vi "RampVoltagewithDDSv6.vi"() -> ()   [LabVIEW 2016]
uses:
  <vilib>/DAQmx/write.llb/DAQmx Write (Digital 1D Wfm NChan NSamp).vi
  <vilib>/DAQmx/write.llb/DAQmx Write (Analog 2D DBL NChan NSamp).vi
  <vilib>/DAQmx/create/channels.llb/DAQmx Create Channel (AO-Voltage-Basic).vi
  <vilib>/Waveform/DWDTOps.llb/DWDT Boolean Array to Digital.vi
  <vilib>/DAQmx/create/channels.llb/DAQmx Create Channel (DO-Digital Output).vi
  <vilib>/DAQmx/configure/timing.llb/DAQmx Timing (Sample Clock).vi
  <vilib>/DAQmx/configure/trigger.llb/DAQmx Start Trigger (Digital Edge).vi
  <vilib>/Waveform/DWDTOps.llb/DWDT Uncompress Digital.vi
  <vilib>/DAQmx/miscellaneous.llb/DAQmx Fill In Error Info.vi
  <vilib>/Waveform/DTblOps.llb/DTbl Digital to Analog.vi
  <resource>/objmgr/daqmx.rc
panel:
  out "Digital Output":cluster{i32, dbl, dbl[][]}(graph)={0, 0.0001, [[5.0, 5.0, 5.0, 5.0, 5.0, 0.0, 0.0, 0.0, 0.0, 0.0, 0.0, 0.0, 0.0, 0.0, 0.0, 0.0, 0.0, 0.0, 0.0, 0.0, 0.0, 0.0, 0.0, 0.0, 0.0, 5.0, 5.0, 5.0, 5.0, 5.0, 5.0, 5.0, 5.0, 5.0, 5.0, 5.0, 5.0, 5.0, 5.0, 5.0, 5.0, 5.0, 5.0, 5.0, 5.0, 0.0, 0.0, 0.0, 0.0, 0.0, 0.0, 0.0, 0.0, 0.0, 0.0, 0.0, 0.0, 0.0, 0.0, 0.0, 0.0, 0.0, 0.0, 0.0, 0.0, 5.0, 5.0, 5.0, 5.0, 5.0], [5.0, 5.0, 5.0, 5.0, 5.0, 0.0, 0.0, 0.0, 0.0, 0.0, 0.0, 0.0, 0.0, 0.0, 0.0, 0.0, 0.0, 0.0, 0.0, 0.0, 0.0, 0.0, 0.0, 0.0, 0.0, 5.0, 5.0, 5.0, 5.0, 5.0, 5.0, 5.0, 5.0, 5.0, 5.0, 5.0, 5.0, 5.0, 5.0, 5.0, 5.0, 5.0, 5.0, 5.0, 5.0, 0.0, 0.0, 0.0, 0.0, 0.0, 0.0, 0.0, 0.0, 0.0, 0.0, 0.0, 0.0, 0.0, 0.0, 0.0, 0.0, 0.0, 0.0, 0.0, 0.0, 5.0, 5.0, 5.0, 5.0, 5.0]]}
  out "Analog Outputs":cluster{i32, dbl, dbl[][]}(graph)={0, 4e-06, array4x1626[6504 elements]}
  in  "High Gain Switch (Port 0 Line 0)":tag="Dev2/port0/line0"
  in  "Ramp to high gain \ndelay (ms)":dbl step=0.01
  in  "error in 2":errorcluster caption="error in"
  in  "ao3 ramp amplitude (V)":dbl=0.4
  in  "ao2 ramp amplitude (V)":dbl=0.3
  in  "ao1 ramp amplitude (V)":dbl=0.2
  in  "SolsTiS 2 - Fast Piezo (ao3)":tag="Dev2/ao3"
  in  "SolsTiS 2 - Slow Piezo (ao2)":tag="Dev2/ao2"
  out "size(s)":i32=1626
  in  "Trigger delay NI (ms)":dbl=0.5
  in  "Trigger Input (PFI0)":tag="/Dev2/PFI0"
  in  "SolsTiS 2 - Fast Piezo (ao1)":tag="Dev2/ao1"
  in  "SolsTiS 1 - Slow Piezo (ao0)":tag="Dev2/ao0"
  in  "Plateau duration (ms)":dbl=2.0 step=0.01
  in  "Ramp duration (ms)":dbl=2.0 step=0.01
  in  "ao0 ramp amplitude (V)":dbl=1.0 step=0.001
  in  "error in":errorcluster
  # "MAGIS LASER SYSTEM\nChirp Control"
  # "Ramp Definition"
  # "Output Monitor"
  # "Channel Definition"
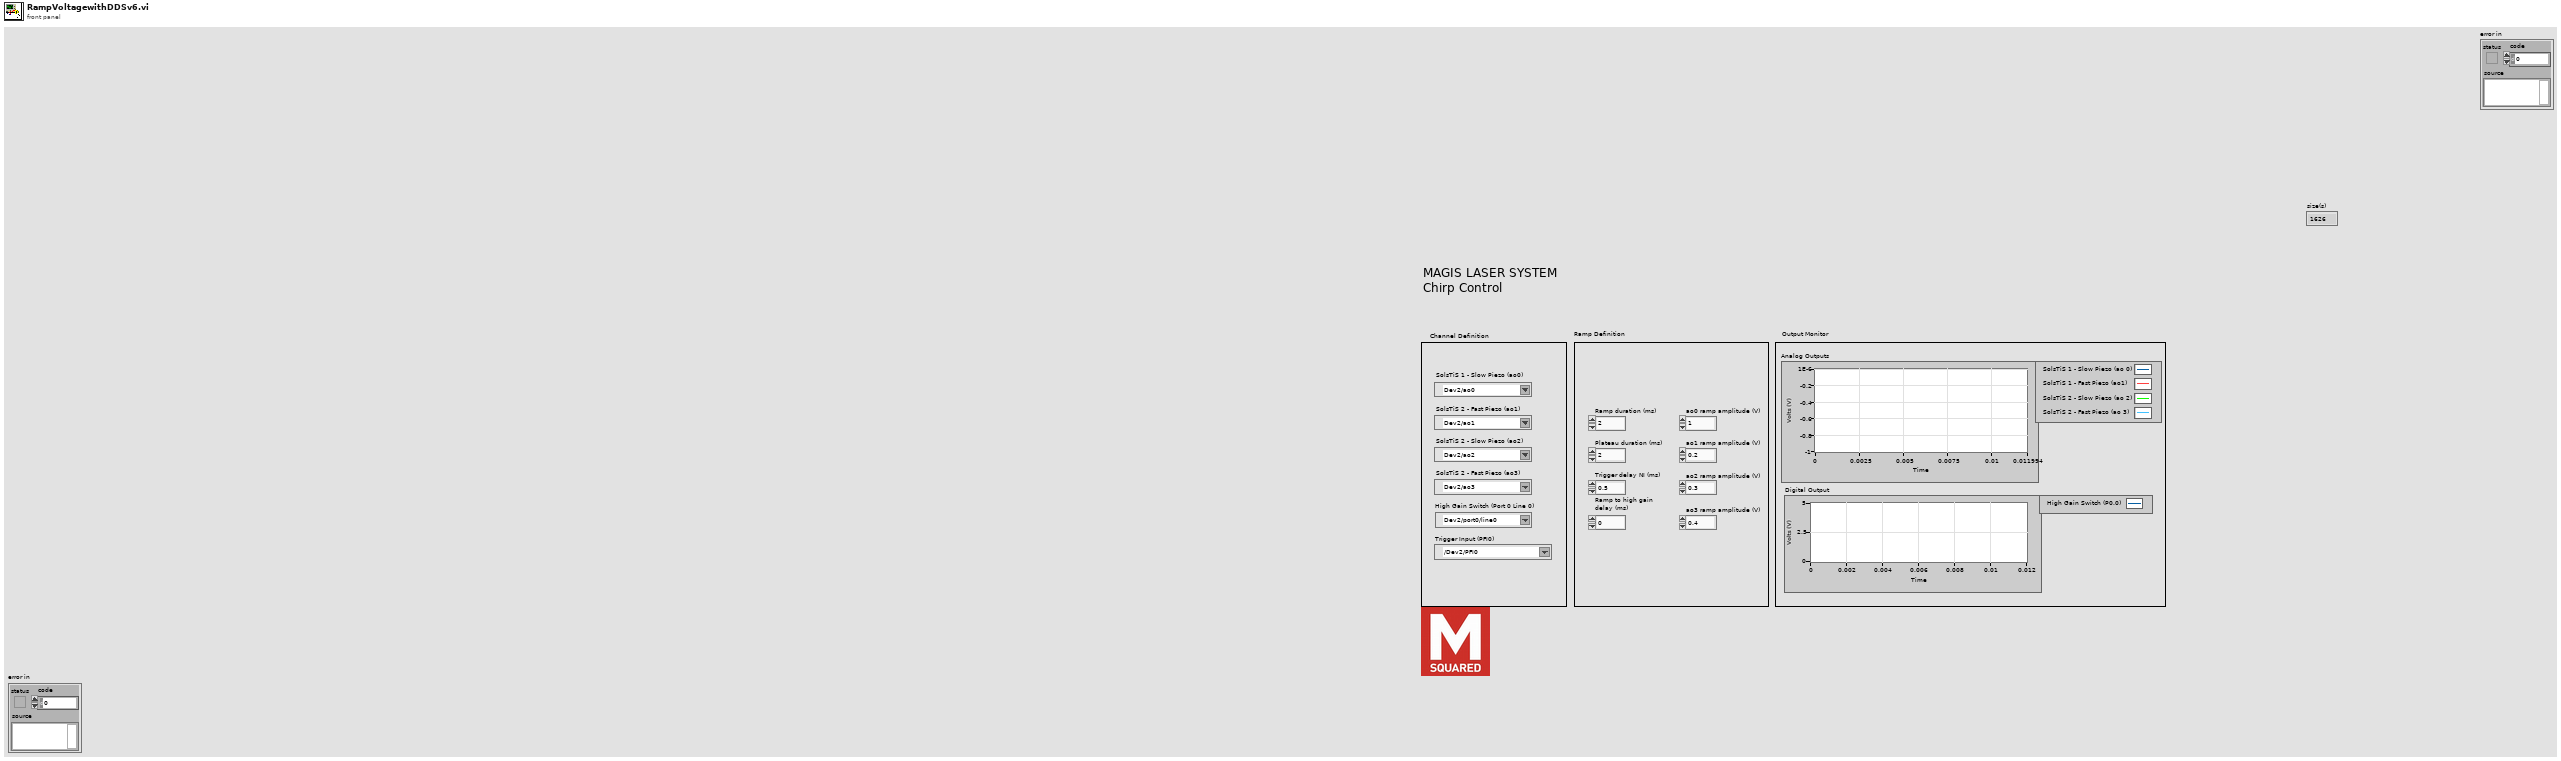
[diagram p1: front panel]
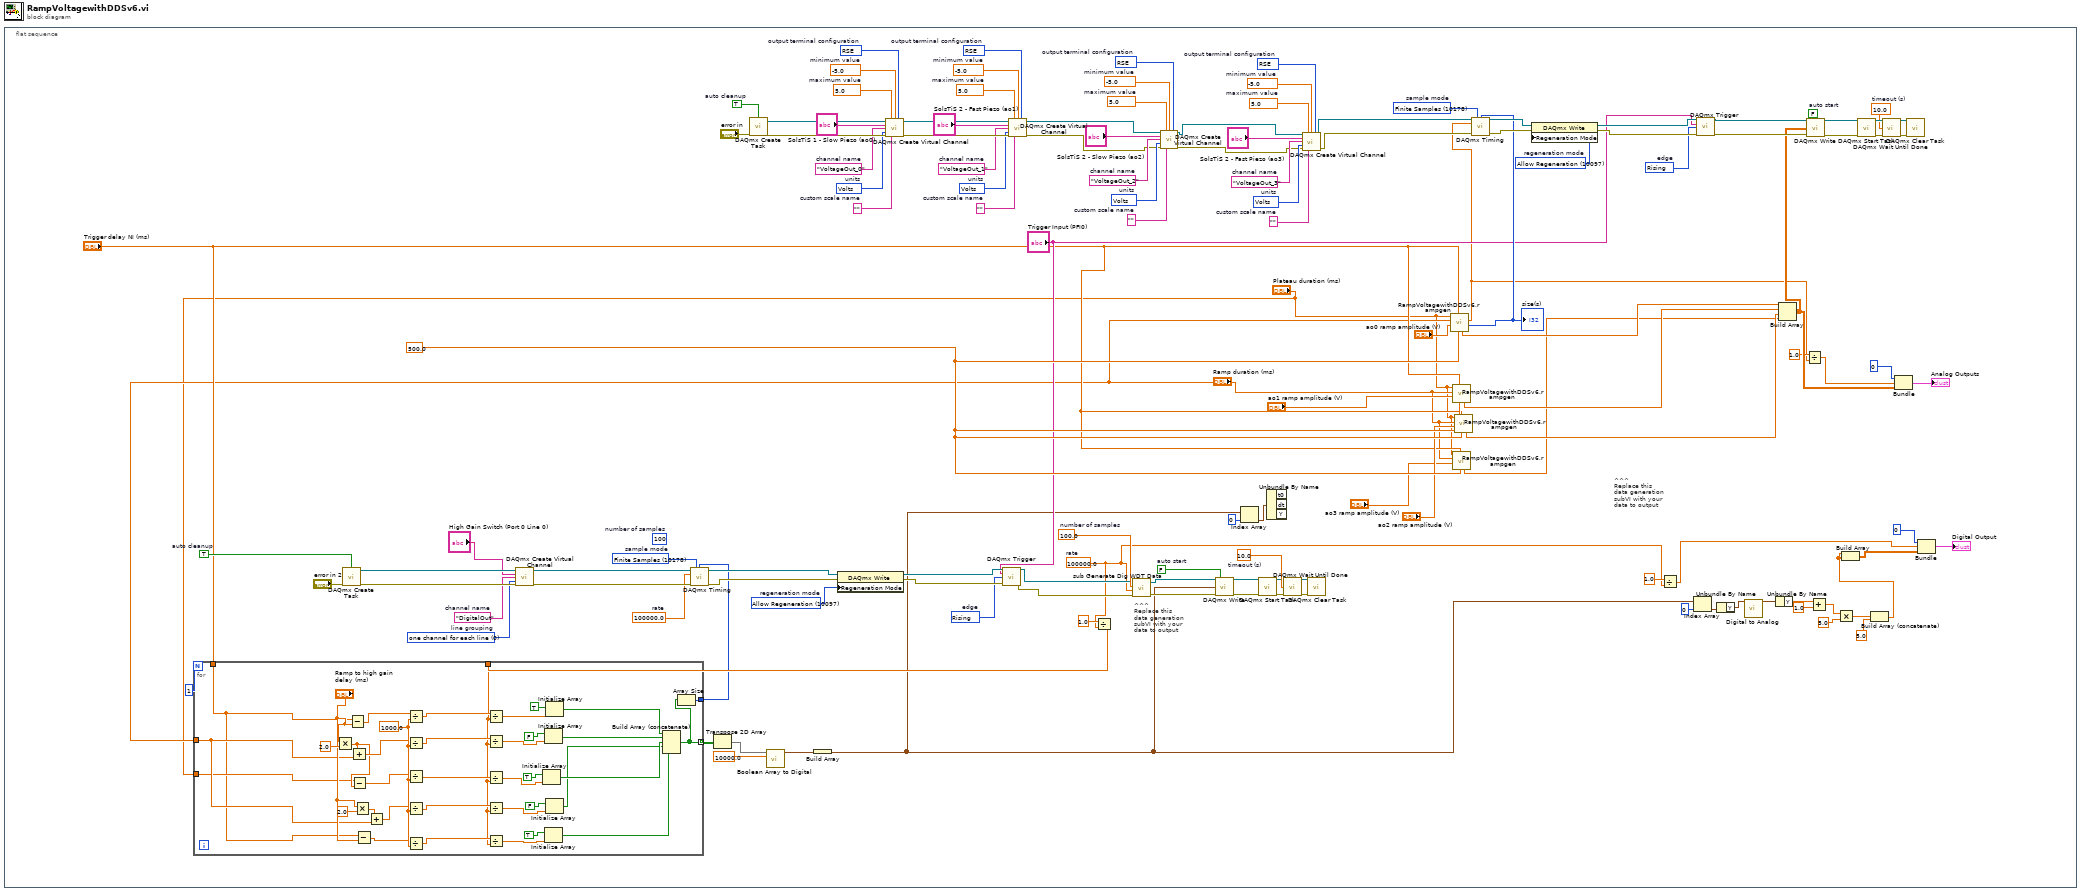
[diagram p0: block diagram]
diagram:
  n1 = flat-sequence {
    frame #0 {
      w75 = 500.0 ("No of samples in ramp (500 or less)")
      w40 = 10280 items=["Rising"=10280, "Falling"=10171]  # edge
      w42 = 10097 items=["Allow Regeneration"=10097, "Do Not Allow Regeneration"=10158]  # regeneration mode
      w45 = 10178 items=["Finite Samples"=10178, "Continuous Samples"=10123, "Hardware Timed Single Point"=12522]  # sample mode
      (unwired) 100  # number of samples
      w46 = 100000.0  # rate
      w51 = 0 items=["one channel for each line", "one channel for all lines"]  # line grouping
      w50 = "DigitalOut"  # channel name
      w53 = TRUE  # auto cleanup
      w68 = 10.0  # timeout (s)
      w9 = 100000.0  # rate
      w61 = 100.0  # number of samples
      w58 = FALSE  # auto start
      w82 = 10083 items=["Default"=-1, "RSE"=10083, "Differential"=10106, "Pseudodifferential"=12529]  # output terminal configuration
      w83 = 10348 items=["Volts"=10348, "From Custom Scale"=10065]  # units
      w84 = "VoltageOut_3"  # channel name
      w85 = ""  # custom scale name
      w86 = -5.0  # minimum value
      w87 = 5.0  # maximum value
      w91 = 10083 items=["Default"=-1, "RSE"=10083, "Differential"=10106, "Pseudodifferential"=12529]  # output terminal configuration
      w92 = 10348 items=["Volts"=10348, "From Custom Scale"=10065]  # units
      w93 = "VoltageOut_2"  # channel name
      w94 = ""  # custom scale name
      w95 = -5.0  # minimum value
      w96 = 5.0  # maximum value
      w103 = 10280 items=["Rising"=10280, "Falling"=10171]  # edge
      w105 = 10097 items=["Allow Regeneration"=10097, "Do Not Allow Regeneration"=10158]  # regeneration mode
      w108 = 10178 items=["Finite Samples"=10178, "Continuous Samples"=10123, "Hardware Timed Single Point"=12522]  # sample mode
      w110 = 10083 items=["Default"=-1, "RSE"=10083, "Differential"=10106, "Pseudodifferential"=12529]  # output terminal configuration
      w111 = 10348 items=["Volts"=10348, "From Custom Scale"=10065]  # units
      w112 = "VoltageOut_1"  # channel name
      w113 = ""  # custom scale name
      w114 = -5.0  # minimum value
      w115 = 5.0  # maximum value
      w117 = 10083 items=["Default"=-1, "RSE"=10083, "Differential"=10106, "Pseudodifferential"=12529]  # output terminal configuration
      w118 = 10348 items=["Volts"=10348, "From Custom Scale"=10065]  # units
      w119 = "VoltageOut_0"  # channel name
      w121 = ""  # custom scale name
      w122 = -5.0  # minimum value
      w123 = 5.0  # maximum value
      w125 = TRUE  # auto cleanup
      w131 = 10.0  # timeout (s)
      w135 = FALSE  # auto start
      # "^^^\nReplace this\ndata generation\nsubVI with your\ndata to output"
      # "^^^\nReplace this\ndata generation\nsubVI with your\ndata to output"
      n2 = call <vilib>:"DAQmx Create Task.vi"("auto cleanup"=w53, "error in"="error in 2") -> ("task out"=w52:refnum<k21>, "error out"=w54:errorcluster)  [unwired: 12 in]
      n3 = call-poly <vilib>:"DAQmx Create Virtual Channel.vi"("task in"=w52, "lines"="High Gain Switch (Port 0 Line 0)", "name to assign"=w50, "line grouping"=w51, "error in"=w54) -> ("task out"=w47:refnum<k21>, "error out"=w49:errorcluster)  [unwired: 9 in]
      n4 = call <vilib>:"DAQmx Create Task.vi"("auto cleanup"=w125, "error in"="error in") -> ("task out"=w124:refnum<k21>, "error out"=w126:errorcluster)  [unwired: 12 in]
      n5 = call-poly <vilib>:"DAQmx Create Virtual Channel.vi"("task in"=w124, "maximum value"=w123, "minimum value"=w122, "output terminal configuration"=w117, "physical channels"="SolsTiS 1 - Slow Piezo (ao0)", "name to assign"=w119, "units"=w118, "error in"=w126, "custom scale name"=w121) -> ("task out"=w116:refnum<k21>, "error out"=w120:errorcluster)  [unwired: 5 in]
      n6 = call-poly <vilib>:"DAQmx Create Virtual Channel.vi"("task in"=w116, "maximum value"=w115, "minimum value"=w114, "output terminal configuration"=w110, "physical channels"="SolsTiS 2 - Fast Piezo (ao1)", "name to assign"=w112, "units"=w111, "error in"=w120, "custom scale name"=w113) -> ("task out"=w89:refnum<k21>, "error out"=w88:errorcluster)  [unwired: 5 in]
      n7 = Divide(x=1.0, y=w9) -> (x/y=w36:dbl)
      n8 = for {
        N: 1 -> [_]
        tunnel: w36 -> [w164]
        tunnel: [w150] -> w33 mode=indexing
        tunnel: [w149] -> w31
        tunnel: "Ramp duration (ms)" -> [w138]
        tunnel: "Plateau duration (ms)" -> [w137]
        tunnel: "Trigger delay NI (ms)" -> [w136]
        w170 = 1000.0
        n9 = Multiply(x="Ramp to high gain \ndelay (ms)", y=2.0) -> (x*y=w145:dbl)
        n10 = Subtract(x=w136, y="Ramp to high gain \ndelay (ms)") -> (x-y=w148:dbl)
        n11 = Add(x=w145, y=w138) -> (x+y=w146:dbl)
        n12 = Subtract(x=w137, y=w145) -> (x-y=w144:dbl)
        n13 = Multiply(x="Ramp to high gain \ndelay (ms)", y=2.0) -> (x*y=w142:dbl)
        n14 = Subtract(x=w136, y="Ramp to high gain \ndelay (ms)") -> (x-y=w139:dbl)
        n15 = Add(x=w142, y=w138) -> (x+y=w141:dbl)
        n16 = Divide(x=w148, y=w170) -> (x/y=w169:dbl)
        n17 = Divide(x=w146, y=w170) -> (x/y=w168:dbl)
        n18 = Divide(x=w144, y=w170) -> (x/y=w167:dbl)
        n19 = Divide(x=w141, y=w170) -> (x/y=w166:dbl)
        n20 = Divide(x=w139, y=w170) -> (x/y=w165:dbl)
        n21 = Divide(x=w169, y=w164) -> (x/y=w160:dbl)
        n22 = Divide(x=w168, y=w164) -> (x/y=w159:dbl)
        n23 = Divide(x=w167, y=w164) -> (x/y=w158:dbl)
        n24 = Divide(x=w166, y=w164) -> (x/y=w157:dbl)
        n25 = Divide(x=w165, y=w164) -> (x/y=w156:dbl)
        n26 = Initialize Array(TRUE, w158) -> (w153:bool[])
        n27 = Initialize Array(FALSE, w159) -> (w154:bool[])
        n28 = Initialize Array(TRUE, w156) -> (w151:bool[])
        n29 = Initialize Array(TRUE, w160) -> (w155:bool[])
        n30 = Initialize Array(FALSE, w157) -> (w152:bool[])
        n31 = Build Array (concatenate)(w155, w154, w153, w152, w151) -> (w150:bool[])
        n32 = Array Size(array=w150) -> (size(s)=w149:i32)
      }
      n33 = call-poly <vilib>:"DAQmx Timing.vi"("task/channels in"=w47, "sample mode"=w45, "samples per channel"=w31, "rate"=w46, "error in"=w49) -> ("task out"=w44:refnum<k21>, "error out"=w48:errorcluster)  [unwired: 9 in]
      n34 = Transpose 2D Array(2D array=w33) -> (transposed array=w34:bool[][])
      n35 = call-poly <vilib>:"Boolean Array to Digital.vi"("sample rate"=10000.0, "boolean array"=w34) -> ("digital waveform"=w32:digitalwaveform)  [unwired: 8 in, 1 out]
      n36 = Build Array(w32) -> (w19:digitalwaveform[])
      n37 = property class="DAQmx Write"(reference=w44, error in=w48, "Regeneration Mode"=w42) -> (reference out=w41:refnum<k21>, error out=w43:errorcluster)
      n38 = call-poly <vilib>:"DAQmx Trigger.vi"("task/channels in"=w41, "source"="Trigger Input (PFI0)", "edge"=w40, "error in"=w43) -> ("task out"=w39:refnum<k21>, "error out"=w38:errorcluster)  [unwired: 10 in]
      n39 = call <vilib>:"sub Generate Dig WDT Data.vi"("task in"=w39, "number of samples"=w61, "update rate"=w9, "error in"=w38) -> ("task out"=w60:refnum<k21>, "error out"=w59:errorcluster)  [unwired: 1 in, 1 out]
      n40 = call-poly <vilib>:"DAQmx Create Virtual Channel.vi"("task in"=w89, "maximum value"=w96, "minimum value"=w95, "output terminal configuration"=w91, "physical channels"="SolsTiS 2 - Slow Piezo (ao2)", "name to assign"=w93, "units"=w92, "error in"=w88, "custom scale name"=w94) -> ("task out"=w80:refnum<k21>, "error out"=w79:errorcluster)  [unwired: 5 in]
      n41 = call-poly <vilib>:"DAQmx Write.vi"("task/channels in"=w60, "auto start"=w58, "data"=w19, "error in"=w59) -> ("task out"=w65:refnum<k21>, "error out"=w66:errorcluster)  [unwired: 9 in, 1 out]
      n42 = Index Array(array=w19, index=0) -> (element=w56:digitalwaveform)
      n43 = call <vilib>:"DAQmx Start Task.vi"("task/channels in"=w65, "error in"=w66) -> ("task out"=w62:refnum<k21>, "error out"=w63:errorcluster)  [unwired: 12 in]
      n44 = Unbundle By Name(w56) -> ()  [unwired: 3 out]
      n45 = call <vilib>:"DAQmx Wait Until Done.vi"("task/channels in"=w62, "timeout (sec)"=w68, "error in"=w63) -> ("task out"=w67:refnum<k21>, "error out"=w64:errorcluster)  [unwired: 11 in]
      n46 = call-poly <vilib>:"DAQmx Create Virtual Channel.vi"("task in"=w80, "maximum value"=w87, "minimum value"=w86, "output terminal configuration"=w82, "physical channels"="SolsTiS 2 - Fast Piezo (ao3)", "name to assign"=w84, "units"=w83, "error in"=w79, "custom scale name"=w85) -> ("task out"=w77:refnum<k21>, "error out"=w78:errorcluster)  [unwired: 5 in]
      n47 = call <vilib>:"DAQmx Clear Task.vi"("task in"=w67, "error in"=w64) -> ()  [unwired: 13 in, 1 out]
      n48 = call "RampVoltagewithDDSv6,rampgen.vi"("No of samples in ramp"=w75, "Trigger delay NI (ms)"="Trigger delay NI (ms)", "Ramp Amplitude (V)}"="ao0 ramp amplitude (V)", "Ramp duration (ms)"="Ramp duration (ms)", "Plateau duration (ms)"="Plateau duration (ms)") -> ("Numeric 2"=w99:i32, "Numeric"=w12:dbl, "Array"=w76:dbl[])  [unwired: 3 in, 1 out]
      "size(s)" <- w99
      n49 = call "RampVoltagewithDDSv6,rampgen.vi"("No of samples in ramp"=w75, "Trigger delay NI (ms)"="Trigger delay NI (ms)", "Ramp Amplitude (V)}"="ao1 ramp amplitude (V)", "Ramp duration (ms)"="Ramp duration (ms)", "Plateau duration (ms)"="Plateau duration (ms)") -> ("Array"=w71:dbl[])  [unwired: 3 in, 3 out]
      n50 = call "RampVoltagewithDDSv6,rampgen.vi"("No of samples in ramp"=w75, "Trigger delay NI (ms)"="Trigger delay NI (ms)", "Ramp Amplitude (V)}"="ao3 ramp amplitude (V)", "Ramp duration (ms)"="Ramp duration (ms)", "Plateau duration (ms)"="Plateau duration (ms)") -> ("Array"=w69:dbl[])  [unwired: 3 in, 3 out]
      n51 = call "RampVoltagewithDDSv6,rampgen.vi"("No of samples in ramp"=w75, "Trigger delay NI (ms)"="Trigger delay NI (ms)", "Ramp Amplitude (V)}"="ao2 ramp amplitude (V)", "Ramp duration (ms)"="Ramp duration (ms)", "Plateau duration (ms)"="Plateau duration (ms)") -> ("Array"=w70:dbl[])  [unwired: 3 in, 3 out]
      n52 = call-poly <vilib>:"DAQmx Timing.vi"("task/channels in"=w77, "sample mode"=w108, "samples per channel"=w99, "rate"=w12, "error in"=w78) -> ("task out"=w107:refnum<k21>, "error out"=w109:errorcluster)  [unwired: 9 in]
      n53 = property class="DAQmx Write"(reference=w107, error in=w109, "Regeneration Mode"=w105) -> (reference out=w104:refnum<k21>, error out=w106:errorcluster)
      n54 = Divide(x=1.0, y=w9) -> (x/y=w8:dbl)
      n55 = Index Array(array=w19, index=0) -> (element=w20:digitalwaveform)
      n56 = call-poly <vilib>:"DAQmx Trigger.vi"("task/channels in"=w104, "source"="Trigger Input (PFI0)", "edge"=w103, "error in"=w106) -> ("task out"=w101:refnum<k21>, "error out"=w100:errorcluster)  [unwired: 10 in]
      n57 = Unbundle By Name(w20) -> ("Y"=w18:digitaldata)
      n58 = call-poly <vilib>:"Digital to Analog.vi"("digital table"=w18) -> ("analog waveform"=w17:waveform(dbl))  [unwired: 7 in, 3 out]
      n59 = Unbundle By Name(w17) -> ("Y"=w6:dbl[])
      n60 = Build Array(w76, w71, w70, w69) -> (w24:dbl[][])
      n61 = Divide(x=1.0, y=w12) -> (x/y=w11:dbl)
      n62 = call-poly <vilib>:"DAQmx Write.vi"("task/channels in"=w101, "auto start"=w135, "data"=w24, "error in"=w100) -> ("task out"=w130:refnum<k21>, "error out"=w129:errorcluster)  [unwired: 9 in, 1 out]
      n63 = Add(x=w6, y=1.0) -> (x+y=w5:dbl[])
      n64 = Multiply(x=w5, y=5.0) -> (x*y=w3:dbl[])
      n65 = call <vilib>:"DAQmx Start Task.vi"("task/channels in"=w130, "error in"=w129) -> ("task out"=w134:refnum<k21>, "error out"=w133:errorcluster)  [unwired: 12 in]
      n66 = Build Array (concatenate)(w3, 5.0 ("y")) -> (w1:dbl[])
      n67 = Build Array(w1, w1) -> (w14:dbl[][])
      n68 = call <vilib>:"DAQmx Wait Until Done.vi"("task/channels in"=w134, "timeout (sec)"=w131, "error in"=w133) -> ("task out"=w128:refnum<k21>, "error out"=w132:errorcluster)  [unwired: 11 in]
      n69 = Bundle(0, w11, w24) -> (→"Analog Outputs":cluster{i32, dbl, dbl[][]})  [unwired: 1 in]
      n70 = call <vilib>:"DAQmx Clear Task.vi"("task in"=w128, "error in"=w132) -> ()  [unwired: 13 in, 1 out]
      n71 = Bundle(0, w8, w14) -> (→"Digital Output":cluster{i32, dbl, dbl[][]})  [unwired: 1 in]
    }
  }
